vi "Convert SNAFU to Decimal.vi"(11 "Cluster":T1) -> (3 "Decimal":i64)   [LabVIEW 2020]
uses:
  Cluster SNAFU Number.ctl
  ENUM_SNAFU Digit.ctl
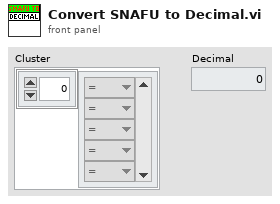
[diagram p1: front panel]
types:
  T1 = typedef "Cluster SNAFU Number.ctl" = cluster{"Digits":T2[]}
  T2 = typedef "ENUM_SNAFU Digit.ctl" = enum16{"=", "-", "0", "1", "2"}
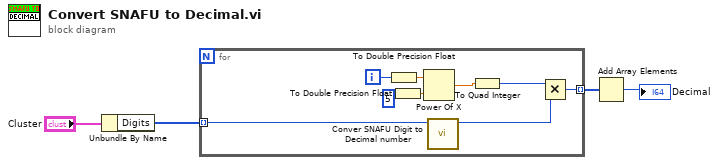
[diagram p0: block diagram]
diagram:
  n1 = Unbundle By Name("Cluster") -> ("Digits"=w1:T2[])
  n2 = for {
    tunnel: w1 -> [w13] mode=indexing
    tunnel: [w11] -> w3 mode=indexing
    i -> [w9]
    n3 = To Double Precision Float(number=w9) -> (double precision float=w8:dbl)
    n4 = To Double Precision Float(number=i64 5) -> (double precision float=w7:dbl)
    n5 = Power Of X(1:w7, 2:w8) -> (0:w6:dbl)
    n6 = call "Conver SNAFU Digit to Decimal number.vi"("SNAFU IDs"=w13) -> ("Decemal"=w12:i64)  [unwired: 10 in]
    n7 = To Quad Integer(1:w6) -> (0:w5:i64)
    n8 = Multiply(x=w5, y=w12) -> (x*y=w11:i64)
  }
  n9 = Add Array Elements(numeric array=w3) -> (sum=→"Decimal":i64)
